vi "Generate RGB U8 values from scaled colour ramps.vi"(5 "Group 2":cluster{"start colour":u32, "end colour":u32}={"start colour"=65280, "end colour"=65535}, 6 "Group 3":cluster{"start colour":u32, "end colour":u32}={"start colour"=255, "end colour"=16711935}, 7 "Group 1":cluster{"start colour":u32, "end colour":u32}={"start colour"=16711680, "end colour"=16776960}, 8 "error in (no error)":errorcluster, 11 "No of Images":i32) -> (0 "error out":errorcluster, 1 "Blue":u8[](array[numeric]), 2 "Green":u8[](array[numeric]), 3 "Red":u8[](array[numeric]))   [LabVIEW 2020]
panel:
  out "Blue":u8
  out "Green":u8
  out "Red":u8
  out "hi(x)":u8
  out "3rd Grouping":i32
  out "2nd Grouping":i32
  out "1st Grouping":i32
  out "x-y*floor(x/y)":i32
  out "floor(x/y)":i32
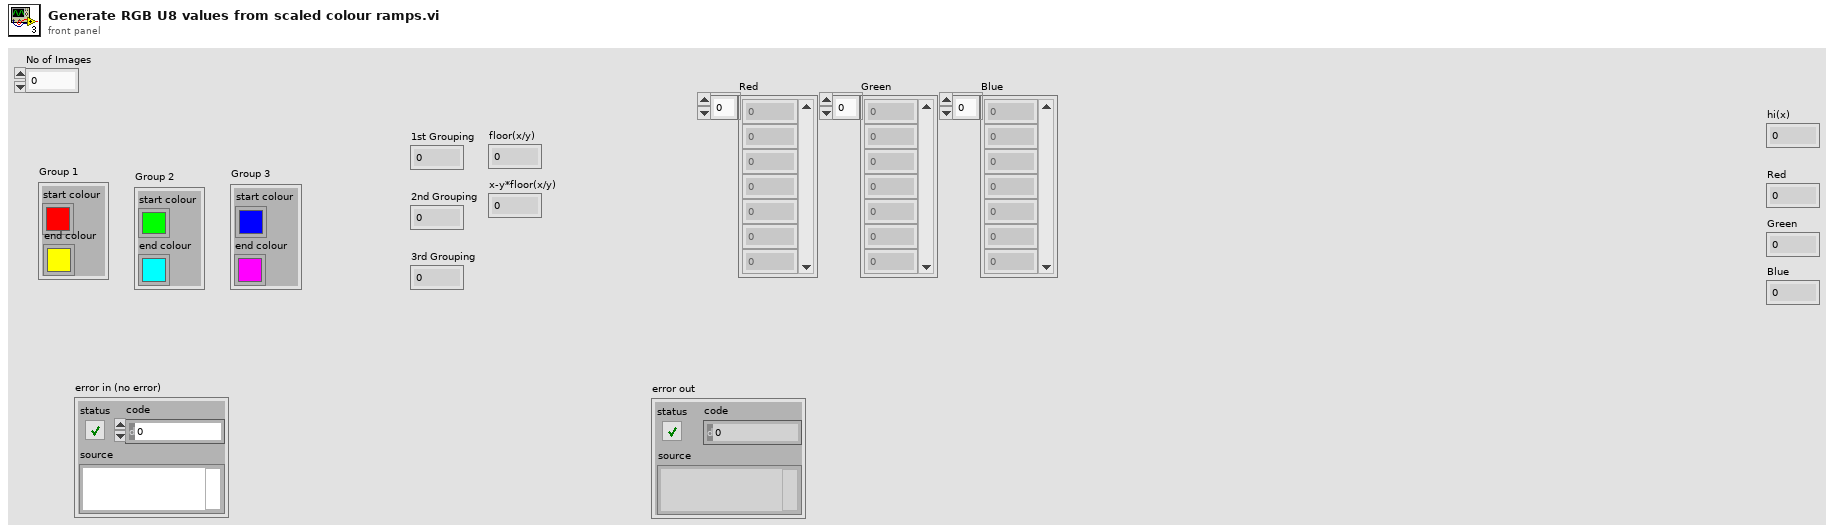
[diagram p1: front panel]
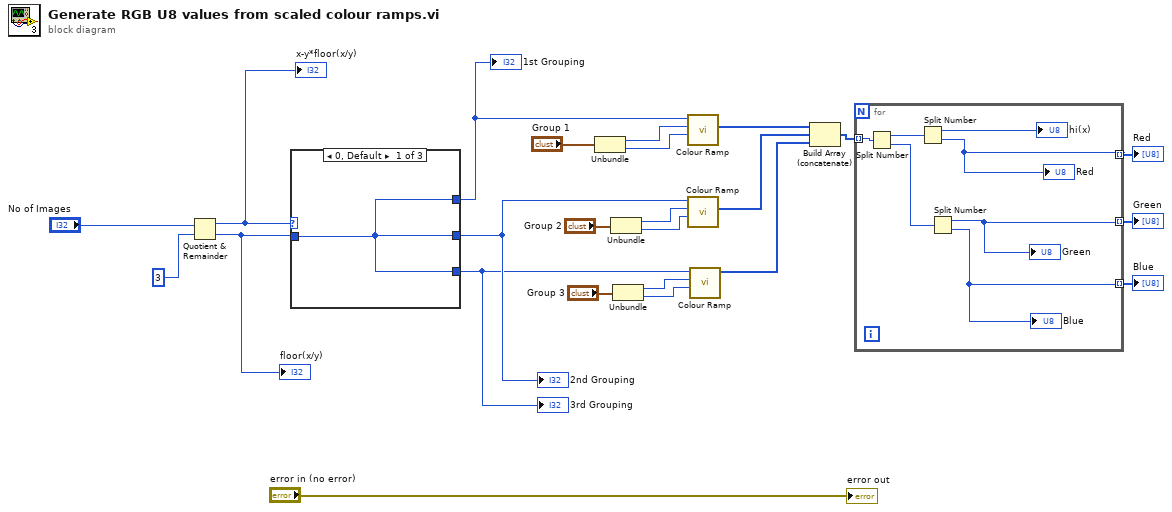
[diagram p0: block diagram]
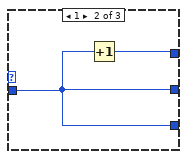
[diagram p2: hidden frame]
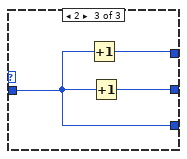
[diagram p3: hidden frame]
diagram:
  n1 = Quotient & Remainder(x="No of Images", y=3) -> (x-y*floor(x/y)=w24:i32, floor(x/y)=w23:i32)
  "floor(x/y)" <- w23
  "x-y*floor(x/y)" <- w24
  n2 = case shown="0, Default" w24 {
    tunnel: w23 -> [w25 w26 w29]
    tunnel: [w25 w27 w30] -> w20
    tunnel: [w25 w26 w28] -> w19
    tunnel: [w25 w26 w29] -> w18
    frame 0, Default {
    }
    frame 1 {
      n3 = Increment(x=w26) -> (x+1=w27:i32)
    }
    frame 2 {
      n4 = Increment(x=w29) -> (x+1=w30:i32)
      n5 = Increment(x=w29) -> (x+1=w28:i32)
    }
  }
  "1st Grouping" <- w20
  "2nd Grouping" <- w19
  "3rd Grouping" <- w18
  n6 = Unbundle("Group 1") -> ("start colour"=w9:u32, "end colour"=w8:u32)
  n7 = Unbundle("Group 2") -> ("start colour"=w6:u32, "end colour"=w5:u32)
  n8 = Unbundle("Group 3") -> ("start colour"=w3:u32, "end colour"=w2:u32)
  n9 = call "Colour Ramp.vi"("End colour"=w8, "Start colour"=w9, "No of colours"=w20) -> ("Colour Array 2"=w17:u32[])  [unwired: 7 in, 1 out]
  n10 = call "Colour Ramp.vi"("End colour"=w5, "Start colour"=w6, "No of colours"=w19) -> ("Colour Array 2"=w16:u32[])  [unwired: 7 in, 1 out]
  n11 = call "Colour Ramp.vi"("End colour"=w2, "Start colour"=w3, "No of colours"=w18) -> ("Colour Array"=w15:u32[])  [unwired: 7 in, 1 out]
  n12 = Build Array (concatenate)(w17, w16, w15) -> (w14:u32[])
  n13 = for {
    tunnel: w14 -> [w34] mode=indexing
    tunnel: [w33] -> w13 mode=indexing
    tunnel: [w32] -> w12 mode=indexing
    tunnel: [w31] -> w11 mode=indexing
    n14 = Split Number(x=w34) -> (hi(x)=w36:u16, lo(x)=w37:u16)
    n15 = Split Number(x=w36) -> (hi(x)=→"hi(x)":u8, lo(x)=w33:u8)
    "Red" <- w33
    n16 = Split Number(x=w37) -> (hi(x)=w32:u8, lo(x)=w31:u8)
    "Green" <- w32
    "Blue" <- w31
  }
  "Red" <- w13
  "Green" <- w12
  "Blue" <- w11
  "error out" <- "error in (no error)"
